vi "CRC8.vi"(1 "DataByte":u8[](array[numeric])) -> (0 "CRC":u8)   [LabVIEW 2013]
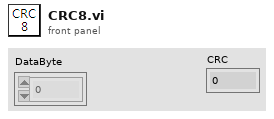
[diagram p1: front panel]
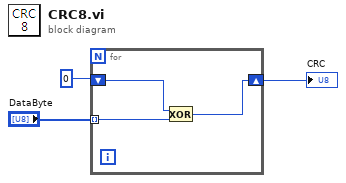
[diagram p0: block diagram]
diagram:
  n1 = for {
    shift-right: [w4] -> w1
    shift-left: u8 0 -> [w6]
    tunnel: "DataByte" -> [w5] mode=indexing
    n2 = Exclusive Or(1:w5, 2:w6) -> (0:w4:u8)
  }
  "CRC" <- w1
